vi "Part 2.vi"(11 "Input":string) -> (3 "Output":i64)   [LabVIEW 2021]
uses:
  <userlib>/_OpenG.lib/string/string.llb/Convert EOLs (String)__ogtk.vi
panel:
  out "Output":bool[][](array[boolean])
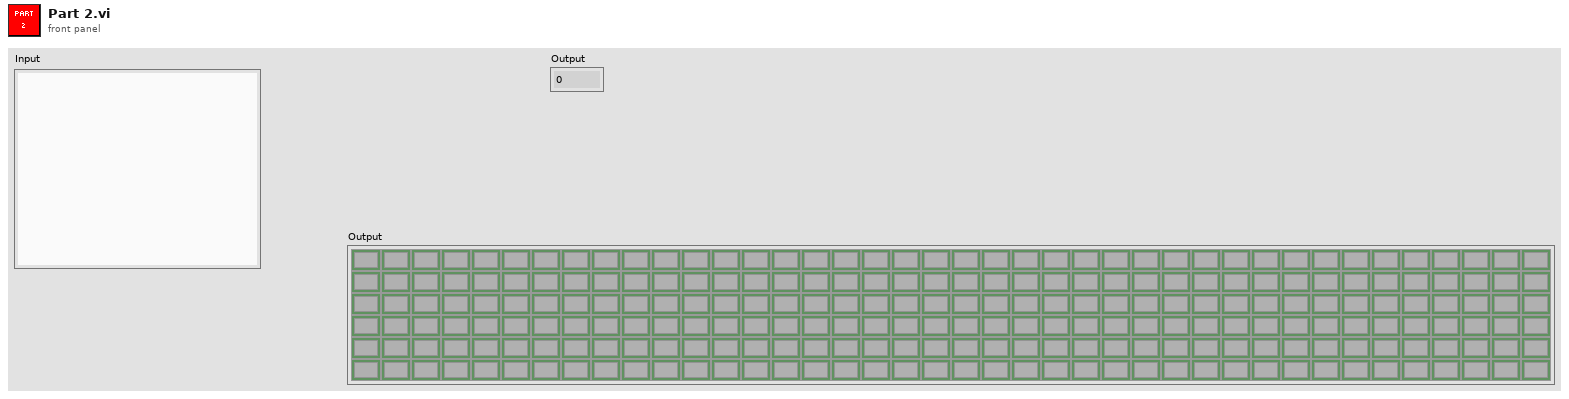
[diagram p1: front panel]
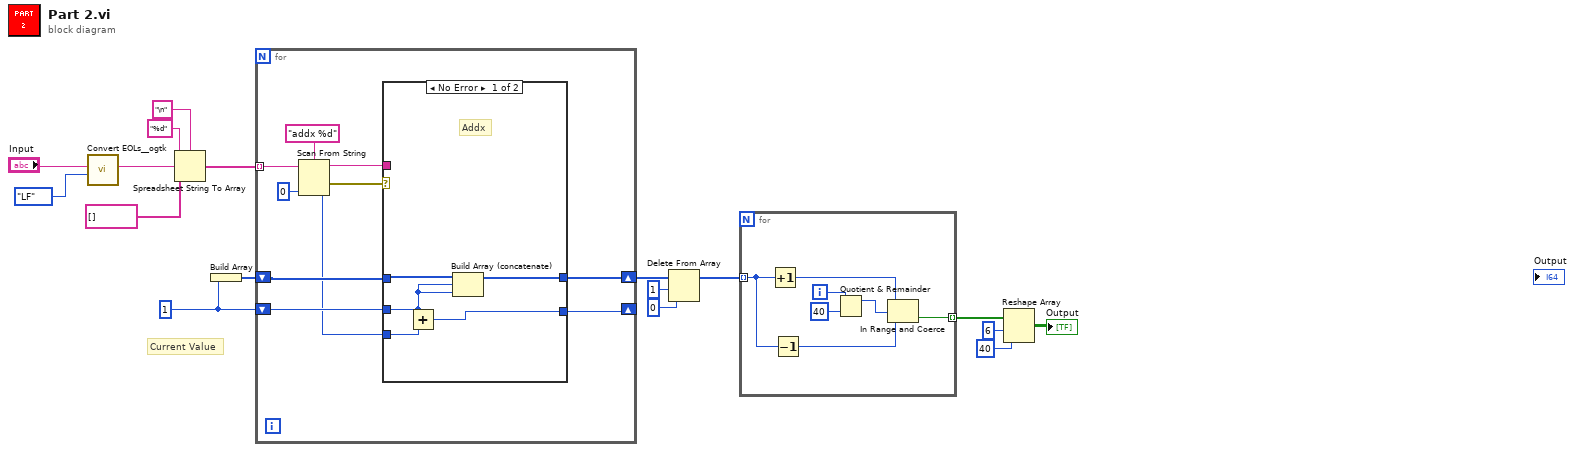
[diagram p0: block diagram]
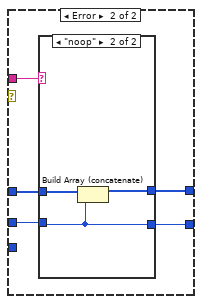
[diagram p2: hidden frame]
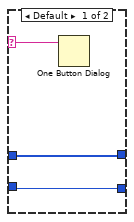
[diagram p3: hidden frame]
diagram:
  w10 = i64 1
  # "Current Value"
  n1 = call-poly <userlib>:"Convert EOLs__ogtk.vi"("Convert to:"=enum16{"CR", "LF", "CRLF"}."LF", "String in"="Input") -> ("String out"=w14:string)  [unwired: 9 in]
  n2 = Spreadsheet String To Array(delimiter (Tab)="\n", format string="%d", spreadsheet string=w14, array type (2D Dbl)=string[] []) -> (array=w12:string[])
  n3 = Build Array(w10) -> (w11:i64[])
  n4 = for {
    tunnel: w12 -> [w27] mode=indexing
    shift-right: [w22] -> w8
    shift-left: w11 -> [w24]
    shift-right: [w21] -> _
    shift-left: w10 -> [w23]
    n5 = Scan From String(format string="addx %d", input string=w27, default 1=i64 0 ("default value 1")) -> (remaining string=w25:string, error out=w26:errorcluster, output 1=w20:i64)  [unwired: 2 in, 1 out]
    n6 = case shown="No Error" w26 {
      tunnel: w25 -> [_ w37]
      tunnel: w24 -> [w29 w36]
      tunnel: w23 -> [w30 w35]
      tunnel: [w28 w34] -> w22
      tunnel: [w31 w33] -> w21
      tunnel: w20 -> [w32 _]
      frame No Error {
        # "Addx"
        n7 = Add(x=w30, y=w32) -> (x+y=w31:i64)
        n8 = Build Array (concatenate)(w29, w30, w30) -> (w28:i64[])
      }
      frame Error {
        n9 = case shown="\"noop\"" w37 {
          selector: w37 -> [w40 _]
          tunnel: w36 -> [w39 w43]
          tunnel: w35 -> [w38 w41]
          tunnel: [w39 w42] -> w34
          tunnel: [w38 w41] -> w33
          frame Default {
            n10 = One Button Dialog(message=w40) -> ()  [unwired: 1 in, 1 out]
          }
          frame "noop" {
            n11 = Build Array (concatenate)(w43, w41) -> (w42:i64[])
          }
        }
      }
    }
  }
  n12 = Delete From Array(array=w8, length=1, index=0) -> (array with subset deleted=w3:i64[])  [unwired: 1 out]
  n13 = for {
    tunnel: w3 -> [w49] mode=indexing
    tunnel: [w47] -> w7 mode=indexing
    i -> [w44]
    n14 = Increment(x=w49) -> (x+1=w50:i64)
    n15 = Decrement(x=w49) -> (x-1=w48:i64)
    n16 = Quotient & Remainder(x=w44, y=40) -> (x-y*floor(x/y)=w45:i32)  [unwired: 1 out]
    n17 = In Range and Coerce(upper limit=w50, x=w45, lower limit=w48) -> (In Range?=w47:bool)  [unwired: 1 out]
  }
  n18 = Reshape Array(w7, 6 ("dimension size"), 40 ("dimension size")) -> (→"Output":bool[][])
